vi "Get Single XML Node By Name.vi"(8 "error in (no error)":errorcluster, 10 "Tag Name":string, 11 "Parent Element":refnum<k20>) -> (0 "error out":errorcluster, 2 "node text":string, 3 "Parent Element Out":refnum<k20>)   [LabVIEW 2013]
uses:
  <vilib>/xml/Close Reference(Node).vi
  <resource>/objmgr/DOMUserDefRef.rc
  <vilib>/xml/NI_XML.lvlib
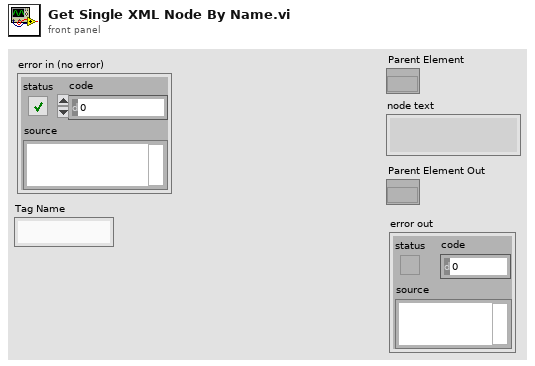
[diagram p1: front panel]
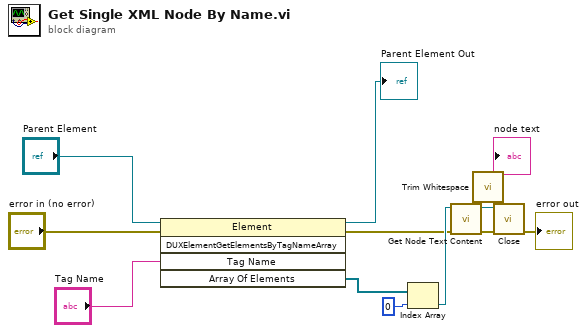
[diagram p0: block diagram]
diagram:
  n1 = invoke class="Element" method="DUXElementGetElementsByTagNameArray"(reference="Parent Element", error in="error in (no error)", "Tag Name"="Tag Name") -> (reference out=→"Parent Element Out":refnum<k20>, error out=w7:errorcluster, "Array Of Elements"=w10:refnum<k20>[])  [unwired: 2 in, 2 out]
  n2 = Index Array(array=w10, index=0) -> (element=w8:refnum<k20>)
  n3 = call <vilib>:"Get Node Text Content.vi"("error in (no error)"=w7, "node in"=w8) -> ("error out"=w4:errorcluster, "node text"=w6:string, "node out"=w5:refnum<k20>)  [unwired: 7 in]
  n4 = call <vilib>:"Trim Whitespace.vi"("string"=w6) -> ("trimmed string"=→"node text":string)  [unwired: 1 in]
  n5 = call-poly <vilib>:"Close.vi"("error in (no error)"=w4, "node"=w5) -> ("error out"=→"error out":errorcluster)  [unwired: 7 in]
